vi "QI_correlation_Y.vi"(6 "拟合半径":i32=5, 11 "QI 传递变量":T1) -> (3 "最相关位置":dbl)   [LabVIEW 2017]
doc: "本VI是QI算法中的核心部分之一，用途在于将x轴上的radial profile 连起来，并和自己的反向做相关性计算，得到相关性曲线后，在最大相关位置附近做二次方程拟合，计算出顶点的坐标，再结合图心坐标做出修正，从而得到小球的xy值，并在下一次测量前修正ROI的位置。\n本VI有一些需要注释的地方，便于后面的调试者理解。\n1、在拼接x轴左边和右边的radial profile前，在中间加了一个0值，这是因为算强度分布的时候没有计算0点的值，如果不补，可能后面会造成坐标的错位，0点的值是不重要的，反正哪个方向的0点值都应该一致，就取默认值即可。\n2、由于相关值算出来比较大，为了简化计算量，对负相关进行了有偏修正，无偏修正的结果似乎很奇怪，不能采用。\n3、拟合半径的设计是基于负相关曲线不是一个单纯的双曲线，由于衍射环有多个亮环，相关曲线也是波浪形，只有对最相关位置的附近做二次拟合才是合适的，对全局拟合的话，其他不是二次分布的点会降低拟合的可信度。拟合半径的默认值是5，应该可以应付大多数情况。\n4、为了达到超越像素的精度，我们直接用拟合的系数计算得到了顶点的x坐标，从而得出最相关位置。\n5、程序框图禁用的部分是调试时使用的显示图之类的，结束调试后应该重新禁用，否则这部分会吃内存并且影响速度。"
uses:
  <vilib>/Analysis/2dsp.llb/1D Cross Correlation (DBL).vi
  <vilib>/Analysis/NI_AALPro.lvlib
panel:
  out "相关曲线":cluster{dbl[], "Best Polynomial Fit":dbl[]}[](graph)
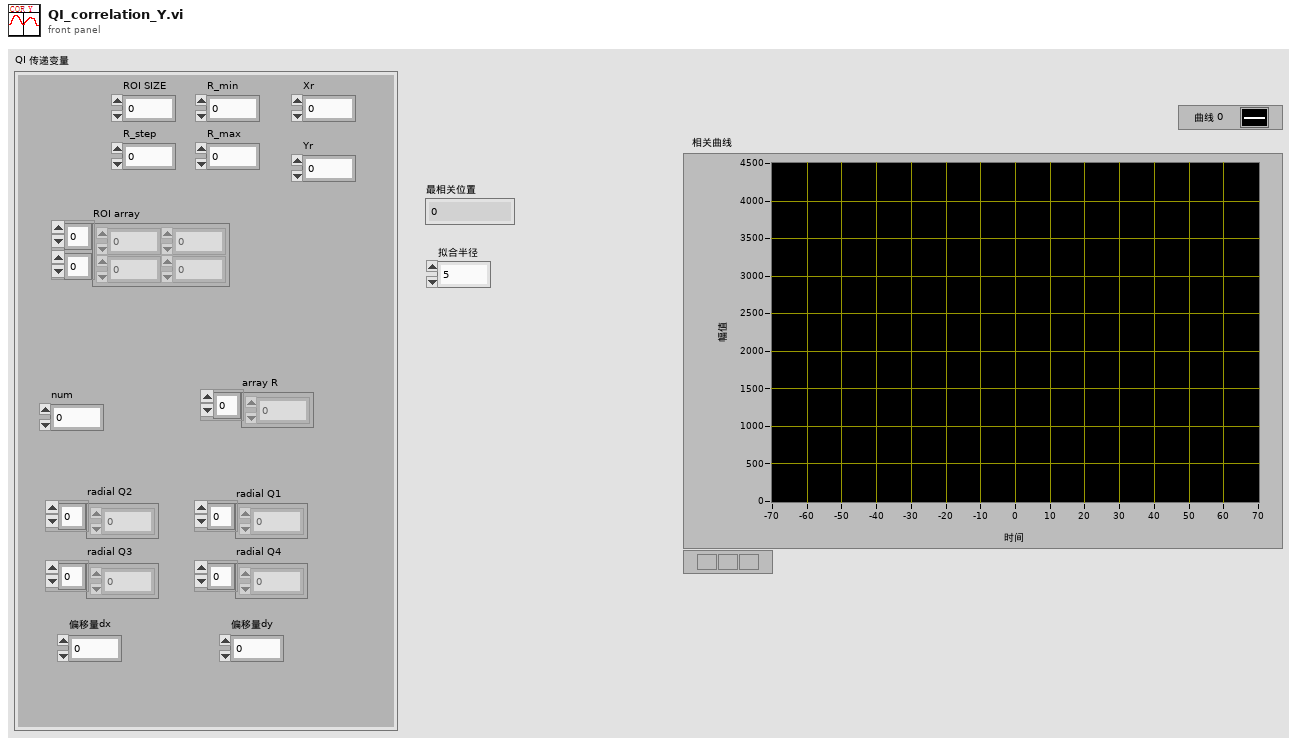
[diagram p1: front panel]
types:
  T1 = typedef "QI 传递变量.ctl" = cluster{"ROI SIZE":i32, "R_step":dbl, "R_min":dbl, "R_max":dbl, "num":dbl, "array R":dbl[], "radial Q1":dbl[], "radial Q2":dbl[], "radial Q3":dbl[], "radial Q4":dbl[], "偏移量dx":dbl, "偏移量dy":dbl, "ROI array":sgl[][], "Xr":dbl, "Yr":dbl}
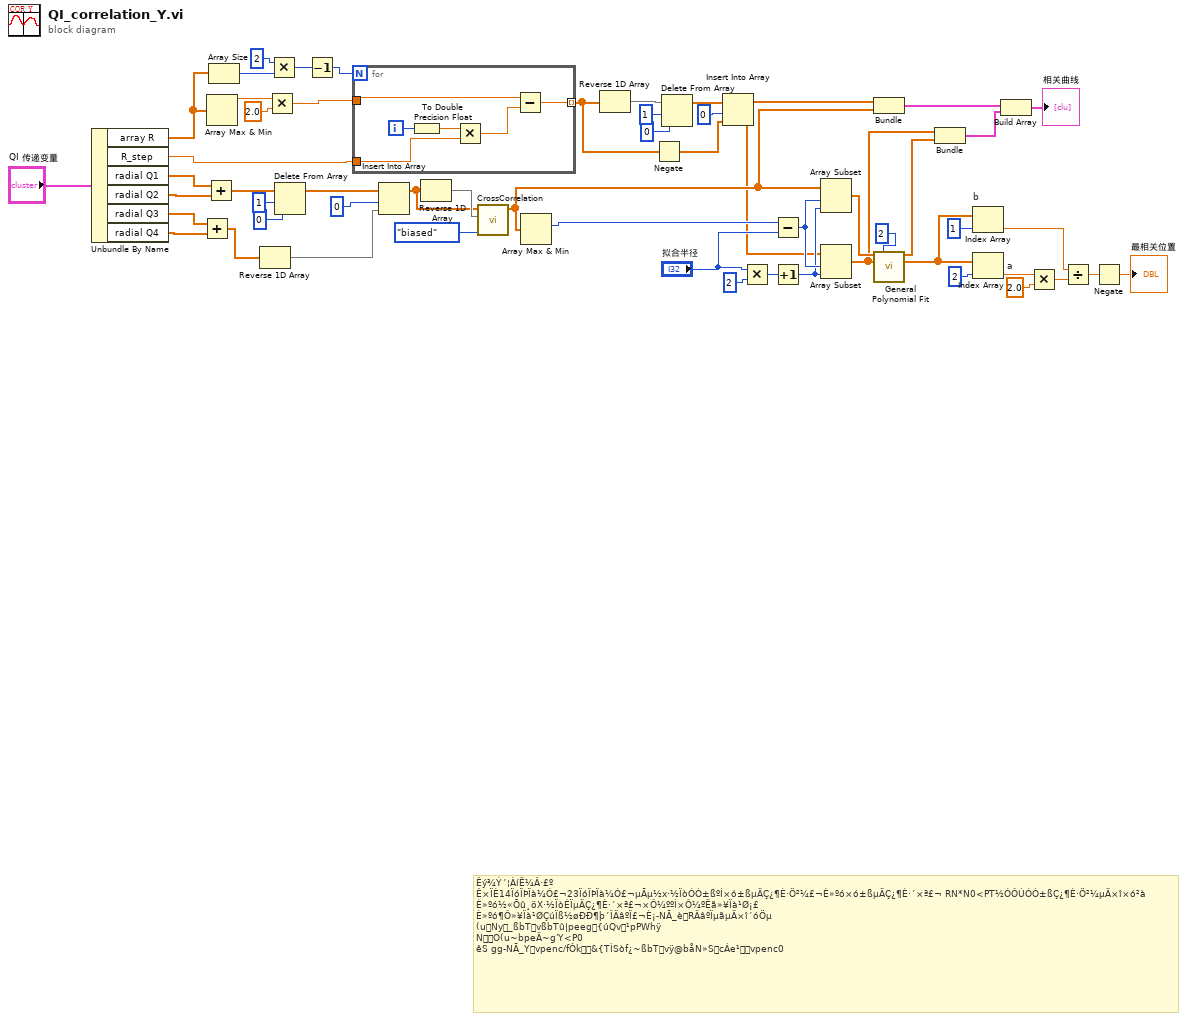
[diagram p0: block diagram]
diagram:
  # "Êý¾Ý´¦ÀíË¼Â·£º\nÊ×ÏÈ14ÏóÏÞÏà¼Ó£¬23ÏóÏÞÏà¼Ó£¬µÃµ½x·½ÏòÓÒ±ßºÍ×ó±ßµÄÇ¿¶È·Ö²¼£¬È»ºó×ó±ßµÄÇ¿¶È·´×ª£¬ RN*N0<PT½ÓÔÚÓÒ±ßÇ¿¶È·Ö²¼µÄ×î×ó²à\nÈ»ºó½«Õû¸öX·½ÏòÉÏµÄÇ¿¶È·´×ª£¬×Ô¼ººÍ×Ô¼ºËã»¥Ïà¹Ø¡£\nÈ»ºó¶Ô»¥Ïà¹ØÇúÏß½øÐÐ¶þ´ÎÄâºÏ£¬È¡-NÃ_èRÄâºÏµãµÄ×î´óÖµ\n(uNy_ßbTvßbTû|peeg{úQv¹pPWhÿ\nNO(u~bpeÄ~g'Y<P0\nêS\tgg-NÃ_Yvpenc/fÔk&{TÌSòf¿~ßbTvÿ@båN»ScÁe¹vpenc0"
  n1 = Unbundle By Name("QI 传递变量") -> ("array R"=w12:dbl[], "R_step"=w11:dbl, "radial Q1"=w52:dbl[], "radial Q2"=w29:dbl[], "radial Q3"=w51:dbl[], "radial Q4"=w28:dbl[])
  n2 = Add(x=w51, y=w28) -> (x+y=w53:dbl[])
  n3 = Add(x=w52, y=w29) -> (x+y=w6:dbl[])
  n4 = Array Max & Min(array=w12) -> (max value=w19:dbl)  [unwired: 3 out]
  n5 = Array Size(array=w12) -> (size(s)=w21:i32)
  n6 = Reverse 1D Array(array=w53) -> (reversed array=w38:dbl[])
  n7 = Multiply(x=w19, y=2.0 ("x")) -> (x*y=w10:dbl)
  n8 = Multiply(x=2, y=w21) -> (x*y=w17:i32)
  n9 = Delete From Array(array=w6, length=1 ("长度"), index=0 ("索引")) -> (array with subset deleted=w5:dbl[])  [unwired: 1 out]
  n10 = Decrement(x=w17) -> (x-1=w9:i32)
  n11 = for "For循环" {
    N: w9 -> [_]
    tunnel: [w61] -> w14 mode=indexing
    tunnel: w11 -> [w59]
    tunnel: w10 -> [w56]
    i -> [w58]
    n12 = To Double Precision Float(number=w58) -> (double precision float=w60:dbl)
    n13 = Multiply(x=w60, y=w59) -> (x*y=w57:dbl)
    n14 = Subtract(x=w56, y=w57) -> (x-y=w61:dbl)
  }
  n15 = Insert Into Array(array=w5, index=0 ("索引"), new element=w38) -> (w34:dbl[])
  n16 = Reverse 1D Array(array=w34) -> (reversed array=w35:dbl[])
  n17 = call-poly <vilib>:"CrossCorrelation.vi"("normalization"=enum32{"none", "unbiased", "biased"}."biased", "Y"=w35, "X"=w34) -> ("Rxy"=w36:dbl[])  [unwired: 7 in, 1 out]
  n18 = Array Max & Min(array=w36) -> (max index (indices)=w33:i32)  [unwired: 3 out]
  n19 = Reverse 1D Array(array=w14) -> (reversed array=w2:dbl[])
  n20 = Negate(x=w14) -> (-x=w15:dbl[])
  n21 = Delete From Array(array=w2, length=1 ("长度"), index=0 ("索引")) -> (array with subset deleted=w1:dbl[])  [unwired: 1 out]
  n22 = Insert Into Array(array=w1, index=0 ("索引"), new element=w15) -> (w13:dbl[])
  n23 = Multiply(x="拟合半径", y=2 ("x")) -> (x*y=w31:i32)
  n24 = Subtract(x=w33, y="拟合半径") -> (x-y=w25:i32)
  n25 = Increment(x=w31) -> (x+1=w24:i32)
  n26 = Array Subset(array=w36, index=w25, length=w24) -> (w39:dbl[])
  n27 = Array Subset(array=w13, index=w25, length=w24) -> (w23:dbl[])
  n28 = Bundle(w13, "Rxy"=w36) -> (w27:cluster{dbl[], "Rxy":dbl[]})  [unwired: 1 in]
  n29 = call <vilib>:"General Polynomial Fit.vi"("Y"=w39, "polynomial order"=2, "X"=w23) -> ("Best Polynomial Fit"=w49:dbl[], "Polynomial Coefficients"=w47:dbl[])  [unwired: 9 in, 2 out]
  n30 = Bundle(w23, "Best Polynomial Fit"=w49) -> (w22:cluster{dbl[], "Best Polynomial Fit":dbl[]})  [unwired: 1 in]
  n31 = Index Array "b"(array=w47, index=1 ("索引")) -> (element=w43:dbl)
  n32 = Index Array "a"(array=w47, index=2 ("索引")) -> (element=w45:dbl)
  n33 = Build Array(w27, w22) -> (→"相关曲线":cluster{dbl[], "Best Polynomial Fit":dbl[]}[])
  n34 = Multiply(x=w45, y=2.0) -> (x*y=w42:dbl)
  n35 = Divide(x=w43, y=w42) -> (x/y=w41:dbl)
  n36 = Negate(x=w41) -> (-x=→"最相关位置":dbl)
